vi "Xbox Buttons Speed Transmission 6740.vi"(0 "A":bool, 5 "B":bool, 7 "Y":bool, 9 "X":bool, 11 "Y in":dbl) -> (10 "Y out":dbl)   [LabVIEW 2019]
panel:
  out "Temp val 2":dbl
  in  "A 2":bool
  in  "B 2":bool
  in  "Y 2":bool
  in  "X 2":bool
  in  "Y in 2":dbl
  out "Y out 2":dbl
  out "Temp val":dbl
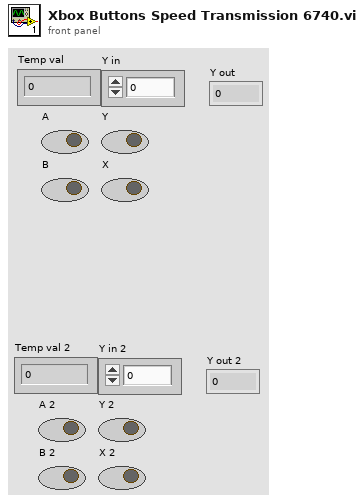
[diagram p1: front panel]
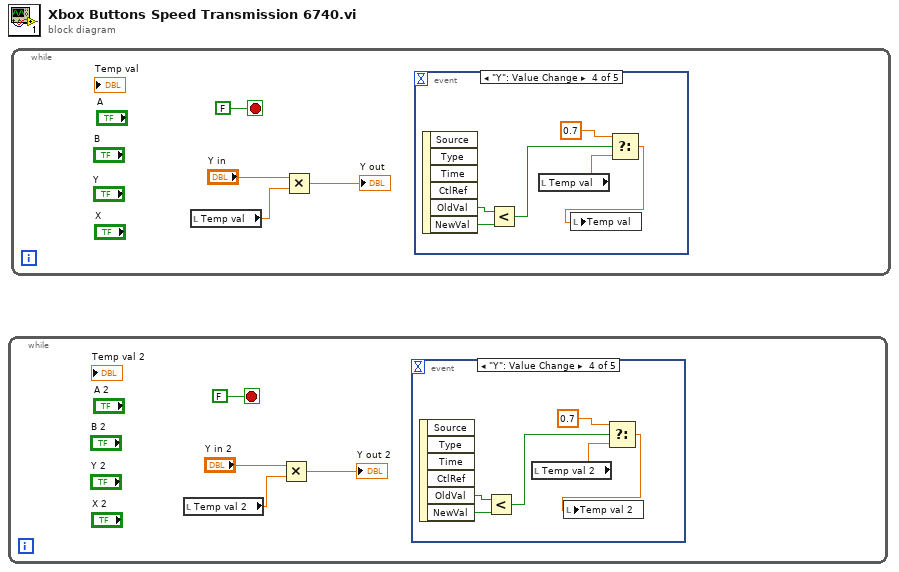
[diagram p0: block diagram]
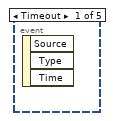
[diagram p2: hidden frame]
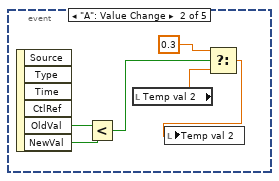
[diagram p3: hidden frame]
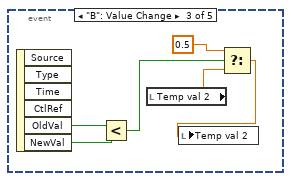
[diagram p4: hidden frame]
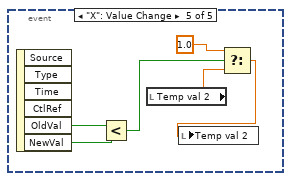
[diagram p5: hidden frame]
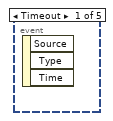
[diagram p6: hidden frame]
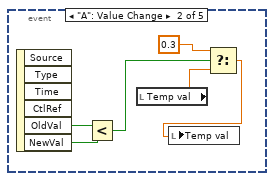
[diagram p7: hidden frame]
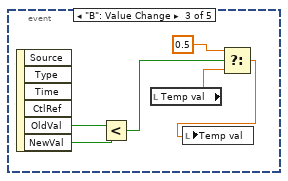
[diagram p8: hidden frame]
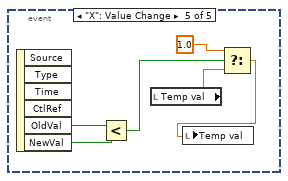
[diagram p9: hidden frame]
diagram:
  n1 = while {
    stop <- FALSE stop-if-true
    n2 = local read "Temp val 2"() -> (w2:dbl)
    n3 = Multiply(x="Y in 2", y=w2) -> (x*y=→"Y out 2":dbl)
    n4 = event shown="[3] \"Y\": Value Change" {
      selector: _ -> [_ _ _ _ _]
      dyn-events: _ -> [_ _ _ _ _]
      timeout: _ -> [_ _ _ _ _]
      event Timeout {
        n5 = event-data() -> ()  [unwired: 1 in, 3 out]
      }
      event "A": Value Change {
        n6 = event-data() -> ("OldVal"=w9:bool, "NewVal"=w10:bool)  [unwired: 1 in, 4 out]
        n7 = Less?(x=w9, y=w10) -> (x < y?=w8:bool)
        n8 = local read "Temp val 2"() -> (w6:dbl)
        n9 = Select(t=0.3 ("Temp val"), s=w8, f=w6) -> (s? t:f=w5:dbl)
        n10 = local write "Temp val 2"(w5) -> ()
      }
      event "B": Value Change {
        n11 = event-data() -> ("OldVal"=w12:bool, "NewVal"=w11:bool)  [unwired: 1 in, 4 out]
        n12 = Less?(x=w12, y=w11) -> (x < y?=w16:bool)
        n13 = local read "Temp val 2"() -> (w14:dbl)
        n14 = Select(t=0.5 ("Temp val"), s=w16, f=w14) -> (s? t:f=w13:dbl)
        n15 = local write "Temp val 2"(w13) -> ()
      }
      event "Y": Value Change {
        n16 = event-data() -> ("OldVal"=w18:bool, "NewVal"=w17:bool)  [unwired: 1 in, 4 out]
        n17 = Less?(x=w18, y=w17) -> (x < y?=w22:bool)
        n18 = local read "Temp val 2"() -> (w20:dbl)
        n19 = Select(t=0.7 ("Temp val"), s=w22, f=w20) -> (s? t:f=w19:dbl)
        n20 = local write "Temp val 2"(w19) -> ()
      }
      event "X": Value Change {
        n21 = event-data() -> ("OldVal"=w24:bool, "NewVal"=w23:bool)  [unwired: 1 in, 4 out]
        n22 = Less?(x=w24, y=w23) -> (x < y?=w28:bool)
        n23 = local read "Temp val 2"() -> (w26:dbl)
        n24 = Select(t=1.0 ("Temp val"), s=w28, f=w26) -> (s? t:f=w25:dbl)
        n25 = local write "Temp val 2"(w25) -> ()
      }
    }
  }
  n26 = while {
    stop <- FALSE stop-if-true
    n27 = local read "Temp val"() -> (w30:dbl)
    n28 = Multiply(x="Y in", y=w30) -> (x*y=→"Y out":dbl)
    n29 = event shown="[3] \"Y\": Value Change" {
      selector: _ -> [_ _ _ _ _]
      dyn-events: _ -> [_ _ _ _ _]
      timeout: _ -> [_ _ _ _ _]
      event Timeout {
        n30 = event-data() -> ()  [unwired: 1 in, 3 out]
      }
      event "A": Value Change {
        n31 = event-data() -> ("OldVal"=w37:bool, "NewVal"=w38:bool)  [unwired: 1 in, 4 out]
        n32 = Less?(x=w37, y=w38) -> (x < y?=w36:bool)
        n33 = local read "Temp val"() -> (w34:dbl)
        n34 = Select(t=0.3 ("Temp val"), s=w36, f=w34) -> (s? t:f=w33:dbl)
        n35 = local write "Temp val"(w33) -> ()
      }
      event "B": Value Change {
        n36 = event-data() -> ("OldVal"=w40:bool, "NewVal"=w39:bool)  [unwired: 1 in, 4 out]
        n37 = Less?(x=w40, y=w39) -> (x < y?=w44:bool)
        n38 = local read "Temp val"() -> (w42:dbl)
        n39 = Select(t=0.5 ("Temp val"), s=w44, f=w42) -> (s? t:f=w41:dbl)
        n40 = local write "Temp val"(w41) -> ()
      }
      event "Y": Value Change {
        n41 = event-data() -> ("OldVal"=w46:bool, "NewVal"=w45:bool)  [unwired: 1 in, 4 out]
        n42 = Less?(x=w46, y=w45) -> (x < y?=w50:bool)
        n43 = local read "Temp val"() -> (w48:dbl)
        n44 = Select(t=0.7 ("Temp val"), s=w50, f=w48) -> (s? t:f=w47:dbl)
        n45 = local write "Temp val"(w47) -> ()
      }
      event "X": Value Change {
        n46 = event-data() -> ("OldVal"=w52:bool, "NewVal"=w51:bool)  [unwired: 1 in, 4 out]
        n47 = Less?(x=w52, y=w51) -> (x < y?=w56:bool)
        n48 = local read "Temp val"() -> (w54:dbl)
        n49 = Select(t=1.0 ("Temp val"), s=w56, f=w54) -> (s? t:f=w53:dbl)
        n50 = local write "Temp val"(w53) -> ()
      }
    }
  }
